vi "Start.vi"(8 "error in (no error)":errorcluster, 11 "AODAcq in":refnum<class "AODAcq.lvclass">) -> (0 "error out":errorcluster, 3 "AODAcq out":refnum<class "AODAcq.lvclass">)   [LabVIEW 2014, in "AODAcq.lvclass"]
uses:
  AODAcq.lvclass
  AODAcq.lvclass/AODAcq.ctl
  <vilib>/Utility/error.llb/Error Cluster From Error Code.vi
  <vilib>/rvi/errors/niLvFpgaAdjustHostInterfaceError.vi
  C:/Program Files (x86)/National Instruments/LabVIEW 2014/Targets/NI/FPGA/StockFPGA_IntfPrivate/ScriptTemplates/StockFPGA_PlugInRead32.vi
  <vilib>/rvi/interface/nirviReadWriteControl/nirviReadWriteControl.xnode
  FPGA_Control/AODRef.ctl
  FPGA Bitfiles/AodScanner_FPGATarget_AODControl(FPGA)_TyJc9yYmyGA.lvbitx
  NiFpgaLv.dll
  <vilib>/FPGAPlugInAG/PXIe-7965R/niLvFpga_Read32_PXIe-7965R.vi
  <vilib>/rvi/interface/nirviReadWriteControl/niFpgaRWControlAccessTimeoutTemplate.vi
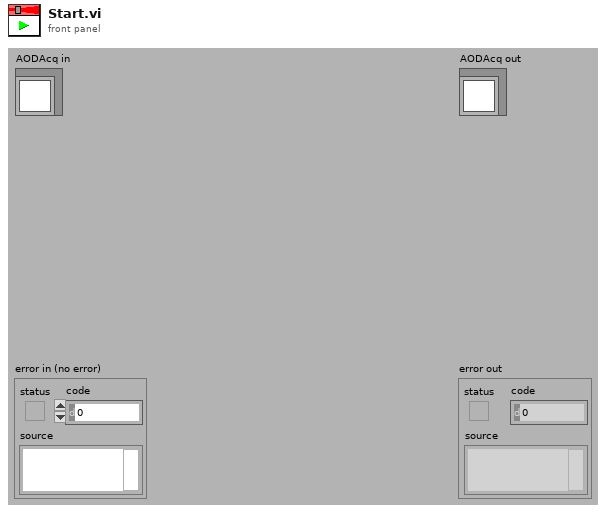
[diagram p1: front panel]
types:
  T1 = typedef "AODRef.ctl" = refnum<k20>
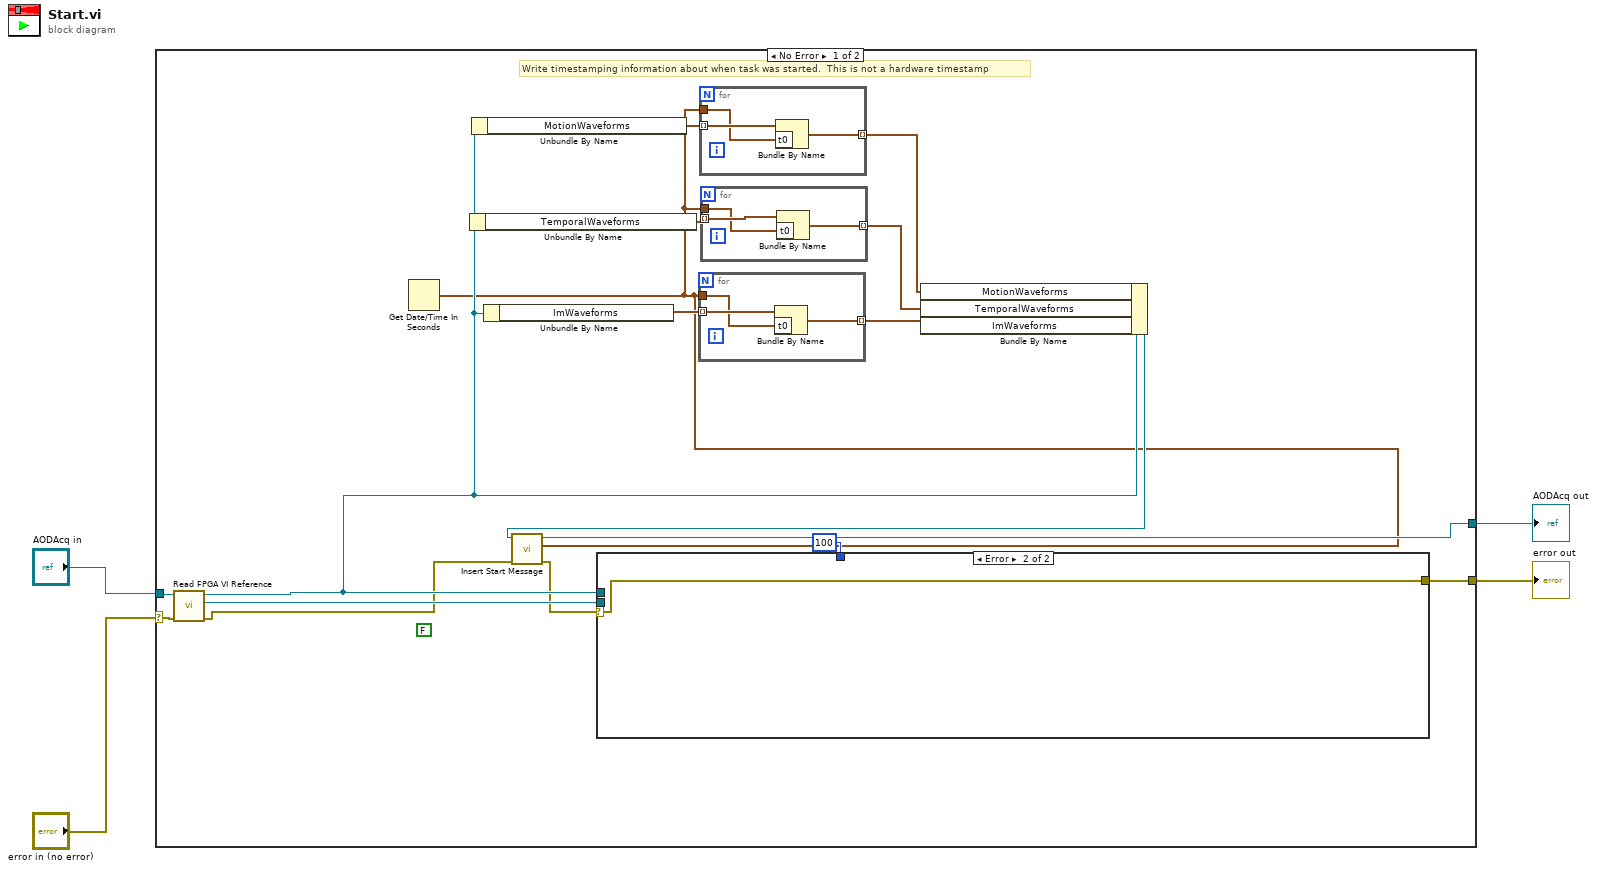
[diagram p0: block diagram]
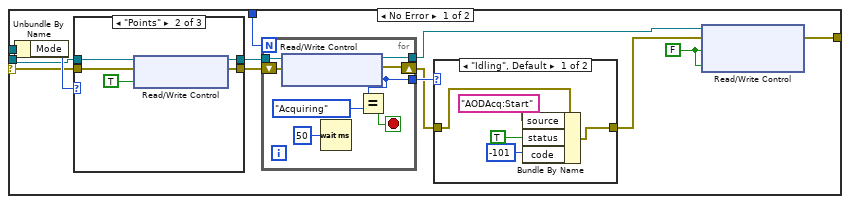
[diagram p2: hidden frame]
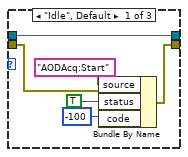
[diagram p4: hidden frame]
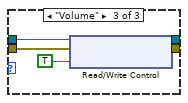
[diagram p5: hidden frame]
diagram:
  n1 = case shown="No Error" "error in (no error)" {
    selector: "error in (no error)" -> [w20 w76]
    tunnel: [w6 w76] -> w3
    tunnel: [w9 w75] -> w1
    tunnel: "AODAcq in" -> [w21 w75]
    frame No Error {
      (unwired) FALSE ("ExtAcqTrig")
      # "Write timestamping information about when task was started.  This is not a hardware timestamp"
      n2 = call-dynamic "Read FPGA VI Reference.vi"("error in (no error)"=w20, "AODAcq in"=w21) -> ("error out"=w7:errorcluster, "FPGA VI Reference"=w11:T1, "AODAcq out"=w12:refnum<class "AODAcq.lvclass">)  [unwired: 7 in]
      n3 = Get Date/Time In Seconds() -> (seconds since 1Jan1904=w8:timestamp)
      n4 = Unbundle By Name(w12) -> ("TemporalWaveforms"=w16:waveform(i32)[])
      n5 = Unbundle By Name(w12) -> ("MotionWaveforms"=w15:waveform(i32)[])
      n6 = Unbundle By Name(w12) -> ("ImWaveforms"=w19:waveform(i32)[])
      n7 = for {
        tunnel: w19 -> [w74] mode=indexing
        tunnel: w8 -> [w73]
        tunnel: [w72] -> w18 mode=indexing
        n8 = Bundle By Name(cluster=w74, "t0"=w73) -> (w72:waveform(i32))
      }
      n9 = for {
        tunnel: w15 -> [w68] mode=indexing
        tunnel: w8 -> [w67]
        tunnel: [w66] -> w13 mode=indexing
        n10 = Bundle By Name(cluster=w68, "t0"=w67) -> (w66:waveform(i32))
      }
      n11 = for {
        tunnel: w16 -> [w71] mode=indexing
        tunnel: w8 -> [w70]
        tunnel: [w69] -> w14 mode=indexing
        n12 = Bundle By Name(cluster=w71, "t0"=w70) -> (w69:waveform(i32))
      }
      n13 = Bundle By Name(cluster=w12, "MotionWaveforms"=w13, "TemporalWaveforms"=w14, "ImWaveforms"=w18) -> (w10:refnum<class "AODAcq.lvclass">)
      n14 = call-dynamic "Insert Start Message.vi"("error in (no error)"=w7, "Start Time"=w8, "AODAcq in"=w10) -> ("error out"=w5:errorcluster, "AODAcq out"=w9:refnum<class "AODAcq.lvclass">)  [unwired: 7 in]
      n15 = case shown="Error" w5 {
        selector: w5 -> [w22 w65]
        tunnel: 100 -> [w33 _]
        tunnel: w12 -> [w30 _]
        tunnel: w11 -> [w28 _]
        tunnel: [w23 w65] -> w6
        frame No Error {
          w29 = FALSE ("ExtAcqTrig")
          n16 = Unbundle By Name(w30) -> ("Mode"=w34:enum16{"Idle", "Points", "Volume"})
          n17 = case shown="\"Points\"" w34 {
            tunnel: w28 -> [w54 w59 w63]
            tunnel: [w54 w58 w62] -> w31
            tunnel: [w50 w56 w61] -> w32
            tunnel: w22 -> [w49 w55 w60]
            frame "Idle", Default {
              n18 = Bundle By Name(cluster=w49, "source"="AODAcq:Start", "status"=TRUE, "code"=-100) -> (w50:errorcluster)
            }
            frame "Points" {
              n19 = xnode "Read/Write Control"("FPGA VI Reference In"=w59, "error in"=w55, "Control.Points"=TRUE) -> ("FPGA VI Reference Out"=w58:T1, "error out"=w56:errorcluster)
            }
            frame "Volume" {
              n20 = xnode "Read/Write Control"("FPGA VI Reference In"=w63, "error in"=w60, "Control.Volume"=TRUE ("Control.Points")) -> ("FPGA VI Reference Out"=w62:T1, "error out"=w61:errorcluster)
            }
          }
          n21 = for {
            N: w33 -> [_]
            tunnel: w31 -> [w48]
            tunnel: [w47] -> w25
            shift-right: [w41] -> w26
            shift-left: w32 -> [w45]
            tunnel: [w42] -> w27
            stop <- w43 stop-if-true
            n22 = xnode "Read/Write Control"("FPGA VI Reference In"=w48, "error in"=w45) -> ("FPGA VI Reference Out"=w47:T1, "error out"=w41:errorcluster, "Status.AcqState"=w42:enum16{"Idling", "Acquiring"})
            n23 = Wait (ms)(milliseconds to wait=u32 50) -> ()  [unwired: 1 out]
            n24 = Equal?(x=w42, y=enum16{"Idling", "Acquiring"}."Acquiring") -> (x = y?=w43:bool)
          }
          n25 = case shown="\"Idling\", Default" w27 {
            tunnel: [w36 w40] -> w24
            tunnel: w26 -> [w35 w40]
            frame "Idling", Default {
              n26 = Bundle By Name(cluster=w35, "source"="AODAcq:Start", "status"=TRUE, "code"=-101) -> (w36:errorcluster)
            }
            frame "Acquiring" {
            }
          }
          n27 = xnode "Read/Write Control"("FPGA VI Reference In"=w25, "error in"=w24, "Control.Points"=w29, "Control.Volume"=w29) -> ("error out"=w23:errorcluster)  [unwired: 1 out]
        }
        frame Error {
        }
      }
    }
    frame Error {
    }
  }
  "error out" <- w3
  "AODAcq out" <- w1
